vi "SLSC Property to Tree Control Item.vi"(9 "string enums":T2(array[cluster]), 10 "Init value":variant, 11 "property":T3) -> (2 "Glyph":i32, 3 "Child Text":string[](array[string]))   [LabVIEW 2017, in "SLSC Tree Control.lvlib"]
doc: "Convert the EDS property datatype to a Tree Control Child Text."
uses:
  SLSC Tree Control.lvlib
  Ctrl/Property.ctl
  Ctrl/EnumValue.ctl
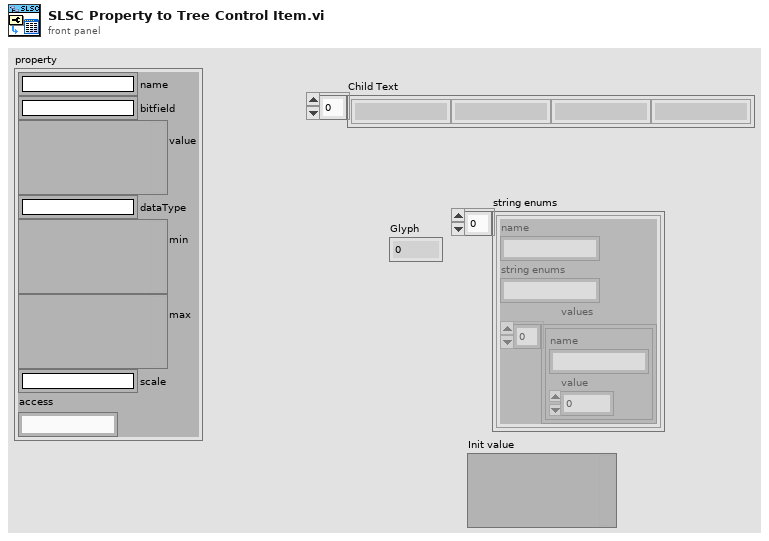
[diagram p1: front panel]
types:
  T1 = typedef "EnumValue.ctl" = cluster{"name":string, "value":i32}
  T2 = cluster{"name":string, "string enums":string, "values":T1[]}[]
  T3 = typedef "Property.ctl" = cluster{"name":string, "bitfield":string, "value":variant, "dataType":string, "min":variant, "max":variant, "scale":string, "access":string}
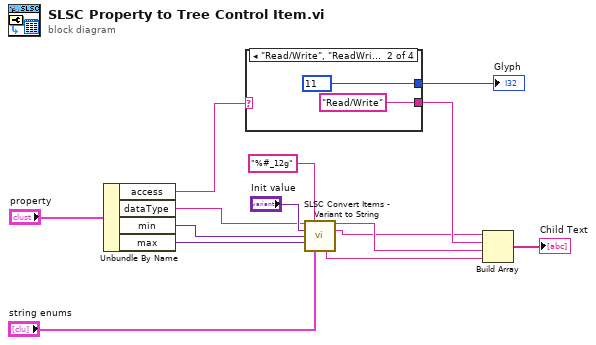
[diagram p0: block diagram]
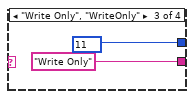
[diagram p3: hidden frame]
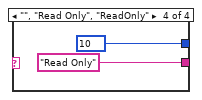
[diagram p4: hidden frame]
diagram:
  n1 = Unbundle By Name("property") -> ("access"=w10:string, "dataType"=w2:string, "min"=w12:variant, "max"=w8:variant)
  n2 = case shown="\"Read/Write\", \"ReadWrite\"" w10 {
    tunnel: [_ "Read/Write" ("string") "Write Only" ("string") "Read Only" ("string")] -> w9
    tunnel: [_ 11 11 10] -> w11
    frame Default {
    }
    frame "Read/Write", "ReadWrite" {
    }
    frame "Write Only", "WriteOnly" {
    }
    frame "", "Read Only", "ReadOnly" {
    }
  }
  "Glyph" <- w11
  n3 = call "SLSC Convert Items - Variant to String.vi"("dataType"=w2, "format string"="%#_12g", "value"="Init value", "min"=w12, "max"=w8, "string enums"="string enums") -> ("Output data type"=w5:string, "string offline data value"=w1:string, "data_range"=w6:string)  [unwired: 5 in, 2 out]
  n4 = Build Array(w1, w9, w5, w6) -> (→"Child Text":string[])
